vi "_Serial Read Bit.vi"(1 "Port type":u8) -> (0 "BitState":bool)   [LabVIEW 2012]
uses:
  <vilib>/eio/EIONode/EIONode.xnode
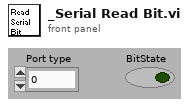
[diagram p1: front panel]
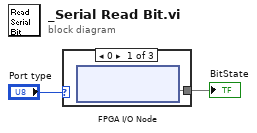
[diagram p0: block diagram]
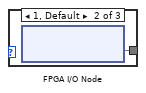
[diagram p2: hidden frame]
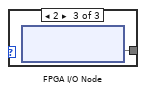
[diagram p3: hidden frame]
diagram:
  n1 = case shown="0" "Port type" {
    tunnel: [w3 w4 w5] -> w2
    frame 0 {
      n2 = xnode "FPGA I/O Node"() -> ("Port5/DIO2"=w3)  [unwired: 1 in, 1 out]
    }
    frame 1, Default {
      n3 = xnode "FPGA I/O Node"() -> ("Port5/DIO0"=w4)  [unwired: 1 in, 1 out]
    }
    frame 2 {
      n4 = xnode "FPGA I/O Node"() -> ("Port6/DIO1"=w5)  [unwired: 1 in, 1 out]
    }
  }
  "BitState" <- w2
